vi "AlliGator Action Loop.vi"(8 "Error In":errorcluster) -> (0 "Error Out":errorcluster)   [LabVIEW 2021, in "AlliGator Action Engine.lvlib"]
doc: "AlliGator action dispatcher.\nEach action array is handled as a package, each action in the array being sent to the appropriate category (Files, Image, Phasor Graph, etc.)."
uses:
  AlliGator Action Engine.lvlib
  Internal Variables/AlliGator Internal Variables v2.ctl
  <vilib>/vision/Image Controls.llb/IMAQ Image.ctl
  Internal Variables/AlliGator Gate Image Set.ctl
  Files/AlliGator FLI Dataset Type.ctl
  Files/AlliGator Data Series Type.ctl
  Dual-Channel Datasets/AlliGator Dataset Channel.ctl
  Settings/AlliGator Gate Arithmetic.ctl
  Source Image/AlliGator Displayed Image.ctl
  Image/Named ROI Description.ctl
  Phasor Graph/AlliGator Decay Metadata v3.ctl
  Decay Analysis/Decay Preprocessing/AlliGator Decay Background Subtraction Info.ctl
  Decay Analysis/Decay Preprocessing/AlliGator Baseline Subtraction Method.ctl
  Graphs/XY Graph/XY Graph Plot Shift Parameters.ctl
  Graphs/XY Graph/XY Graph Plot Shift Method.ctl
  Decay Analysis/Decay Preprocessing/AlliGator Decay Extrapolation Parameters.ctl
  Phasor/Calibration Phasor (m, phi).ctl
  Phasor/Phasor Reference Series.ctl
  Phasor/Phasor Calibration Map v2.ctl
  Phasor/Phasor (g, s).ctl
  Phasor Graph/AlliGator Raw Phasor Plot Data v5.ctl
  Phasor/Phasor Standard Deviation Options.ctl
  Phasor Plot/AlliGator Phasor Multi-Harmonic Data.ctl
  Phasor/Phasor Harmonic Data.ctl
  Decay Fit Parameter Map/AlliGator Decay Fit Options & Parameters v4.ctl
  Fits/IRF(X)PSED/Decay Fit Options v4.ctl
  Fits/Decay Convolution/Decay Model.ctl
  Fits/Residual Type.ctl
  Fits/IRF(X)PSED/Fit Weights Type v2.ctl
  Fits/Non-linear Fitting Method v2.ctl
  Fits/Fit Calculation Method.ctl
  Fits/Non-linear Fitting Algorithm.ctl
  Decay Analysis/Decay Fit/AlliGator Decay Fit Parameter Constraints 2.ctl
  Fits/IRF(X)PSED/Decay Fit Parameters In List.ctl
  Fits/IRF(X)PSED/MLE Baseline Offset Type.ctl
  Decay Analysis/Decay Preprocessing/AlliGator Decay Preprocessing Parameters.ctl
  Fits/IRF(X)PSED/Decay Fit Parameters & Derived Quantities List v2.ctl
  Fits/IRF(X)PSED/Decay Fit Result Constraint.ctl
  Decay Fit Parameter Map/AlliGator Parameter Maps Data.ctl
  Globals, Variables, Constants/AlliGator Refnums List.ctl
  AlliGator Q Event.ctl
  Settings/AlliGator Settings List.ctl
  Graphs/XY Graph/XY Graph Selected Plot Info.ctl
  Graphs/XY Graph/XY Graph Refnum.ctl
  <vilib>/Utility/miscctls.llb/LVPoint32TypeDef.ctl
  Graphs/XY Graph/XY Graph Mouse Click Event Data.ctl
  Debug/AlliGator Debug Action List.ctl
  Alligator Elements Order in Action Stack.ctl
  bb653f8f-7323-4417-bc10-ef5a2241dee5.vi
  Globals, Variables, Constants/AlliGator Globals.vi
  Variant/Variant to Data/Variant to Boolean.vi
  AlliGator Add Action Array to Stack.vi
  Error/Error.lvlib
  Utilities/Utilities.lvlib
  GUI/AlliGator GUI.lvlib
  Notebook/Notebook.lvlib
  Globals, Variables, Constants/AlliGator Globals, Variables & Constants.lvlib
  Settings/AlliGator Settings.lvlib
  Graphs/XY Graph/XY Graph Add-Ons.lvlib
  Variant/Variant to Data/Variant to Data.lvlib
  Decay Fit Parameter Map/AlliGator Decay Fit Parameter Map.lvlib
  Debug/AlliGator Debug.lvlib
  Phasor/Phasor.lvlib
  Image/Image.lvlib
  Decay Analysis/Decay Preprocessing/AlliGator Decay Preprocessing.lvlib
  Phasor Graph/AlliGator Phasor Graph.lvlib
  Files/AlliGator Files.lvlib
  Internal Variables/AlliGator Internal Variables.lvlib
  Phasor Plot/AlliGator Phasor Plot.lvlib
  Source Image/AlliGator Source Image.lvlib
  Fits/Fits.lvlib
  Decay Analysis/Decay Fit/AlliGator Decay Fit.lvlib
  Python Plugins API/AlliGator Python Plugins.lvlib
  Dual-Channel Datasets/AlliGator Dual-Channel Datasets.lvlib
  Test Suites/AlliGator Test Suite.lvlib
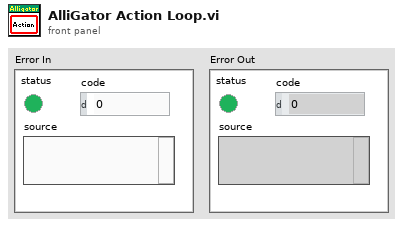
[diagram p1: front panel]
types:
  T1 = typedef "AlliGator Globals, Variables & Constants.lvlib/AlliGator Refnums List.ctl" = enum16{"---------- AlliGator Controls ----------", "AlliGator Tab Control Refnum", "---------- AlliGator Indicators ----------", "Source Image Display Refnum", "Phasor Plot Display Refnum", "Decay Fit Parameter Map Refnum", "---------- AlliGator VIs ----------", "AlliGator Refnum", "AlliGator Settings Refnum", "AlliGator Launcher Refnum"}
  T2 = typedef "AlliGator Internal Variables.lvlib/AlliGator Internal Variables v2.ctl" = cluster{"----------------------------- Images -----------------------------":u8, "Displayed Image":T3, "White Light Image":T3, "Mask Image":T3, "ROI Mask Image":T3, "Current Dataset Images 1":T4, "Background Dataset Images 1":T4, "Current Dataset Images 2":T4, "Background Dataset Images 2":T4, "Current Dataset Arithmetic Images":T4, "Accumulated Dataset Images 1":T4, "Accumulated Dataset Images 2":T4, "Accumulated Dataset Arithmetic Images":T4, "----------------------------- File Paths -----------------------------":u8, "Phasor Plot Image":T3, "Decay Fit Parameter Map Image":T3, "Parameter Map Image":T3, "Single Data Point Path":path, "White Light Image Path":path, "Mask Image Path":path, "Time-Series Folder":path, "[Time-Series Paths]":path[], "----------------------------- FLI Dataset -----------------------------":u8, "Current Dataset":i32, "Single Dataset Type":T5, "Current Folder":string, "AlliGator Data Series Type":T6, "# Datasets":i32, "Dual-Channel Dataset":bool, "Selected Channel Name":string, "Dataset Channel":T7, "Channel Arithmetic":T8, "Dual-Channel Background Dataset":bool, "Background Channel":T7, "Dual-Channel Accumulated Dataset":bool, "Start Time":dbl, "[Time-Series Timestamps]":dbl[], "[Intensity Corrections]":dbl[], "Time Series Script":bool, "Type of Displayed Image":T9, "Gate Image Slide":u16, "# Gates":i32, "ROIs":T10[], "----------------------------- Decays -----------------------------":u8, "ROI Decay":cluster{"t Array":dbl[], "I Array":dbl[]}, "Valid Decay":bool, "Decay  Metadata":T12, "Reference Decay Plot Name":string, "Reference Decay":cluster{"t Array":dbl[], "I Array":dbl[]}, "Decay Shift Plot":cluster{"Time Stamps":dbl[], "Decay Shifts":dbl[]}, "[Decays Max Values]":sgl[], "[Decays Min Values]":sgl[], "----------------------------- Calibration -----------------------------":u8, "Calibration Phasor":T18, "Calibration Phasor Series":T19, "Phasor Calibration Map":T20, "Calibration Map MD5 Digest":string, "----------------------------- Phasor Graph -----------------------------":u8, "Last Raw Phasor":T21, "Last Calibrated Phasor":T21, "Last Calibrated Phasor SDV":T21, "Phasor Graph:Phasor Plot":cluster{"g Array":dbl[], "s Array":dbl[]}, "Phasor Graph:Phasor SDV Plot":cluster{"g Array":dbl[], "s Array":dbl[]}, "[Phasor Graph:Raw Phasor Plots]":T22[], "Phasor Plot locked to Ref 1":i32, "[Phasor Plot(s) locked to Ref 1]":i32[], "[Phasor Plot(s) locked to Ref 2]":i32[], "[Pixel Phasors]":T21[], "----------------------------- Phasor Plot -----------------------------":u8, "[[Sum Image]]":dbl[][], "[[CSG Phasors]]":csg[][], "[[Valid Pixel?]]":bool[][], "[[Phasor Ratios]]":dbl[][], "[[Average Lifetimes]]":dbl[][], "Amplitude Weighted Average Lifetime":bool, "I/m/phi Dataset":cluster{"I/m/phi Dataset?":bool, "Base Frequency":dbl[unit], "Harmonic Orders":u8[]}, "Multi Phasor Plot Data":T24, "----------------------------- Decay Fit Parameter Map -----------------------------":u8, "Decay Fit Options & Parameters":T26, "Fit Options: Decay Preprocessing Parameters":T37, "Fit Options: Reference Decay":cluster{"t Array":dbl[], "I Array":dbl[]}, "Is Full Image Parameters Map":bool, "Is Single-Pixels Parameters Map":bool, "NLSF Parameters Map X Resolution":i32, "NLSF Parameters Map Y Resolution":i32, "[Single Decay Fit Parameters]":dbl[], "Fit Model":T28, "[[Multiple Decays Fit Parameters]]":dbl[][], "[[Multiple Decays Fit Parameter SDVs]]":dbl[][], "[[IRFs]]":dbl[][], "[ROI Descriptors]":T11[], "IRF Array Time Axis":dbl[], "Decay Array Time Axis":dbl[], "[Decay Fit Parameter Names]":T38[], "[Decay Sum]":dbl[], "Array of Decay Fit Result Constraints":T39[], "Selected ROIs Array":bool[], "----------------------------- Parameter Maps -----------------------------":u8, "[Map Set Names]":string[], "[Parameter Maps]":T40[], "[[User-defined Quantities]]":dbl[][], "User-defined Quantity":string}
  T3 = typedef "IMAQ Image.ctl" = refnum<image>
  T4 = typedef "AlliGator Internal Variables.lvlib/AlliGator Gate Image Set.ctl" = cluster{"SGL Gate Images":T3[], "SGL Sum Image":T3, "SGL Max Image":T3, "SGL Min Image":T3}
  T5 = typedef "AlliGator Files.lvlib/AlliGator FLI Dataset Type.ctl" = enum16{"HDF5 FLI Dataset", "Gate Image Folder", ".sdt FLI Dataset (Becker & Hickl)", ".ptu FLI Dataset (PicoQuant)", "SS1 FLI Dataset", "SS2 FLI Dataset", "I/m/phi Dataset", ".bin FLI Dataset (PicoQuant Binned)", ".bin FLI Dataset (Piccolo Binned)", ".mat FLI Dataset"}
  T6 = typedef "AlliGator Files.lvlib/AlliGator Data Series Type.ctl" = enum16{"Not a Supported Series", "Gate Images Folder Series", "SwissSPAD 2 Dataset Series", "B&H FLI Dataset Series", "PicoQuant PTU FLI Dataset Series", "PicoQuant BIN FLI Dataset Series", "Piccolo hist BIN FLI Dataset Series", "HDF5 FLI Dataset Series"}
  T7 = typedef "AlliGator Dual-Channel Datasets.lvlib/AlliGator Dataset Channel.ctl" = enum16{"G2", "INT"}
  T8 = typedef "AlliGator Settings.lvlib/AlliGator Gate Arithmetic.ctl" = enum16{"None", "INT-G2", "G2/INT*<INT>", "(1 - G2/INT)*<INT>"}
  T9 = typedef "AlliGator Source Image.lvlib/AlliGator Displayed Image.ctl" = enum16{"Single Gate", "Sum of All Gates", "Max of All Gates", "Min of All Gates", "-", "White Ligth Image", "Mask Image"}
  T10 = typedef "Image.lvlib/Named ROI Description.ctl" = cluster{"ROI Descriptor":T11, "ROI Name":string, "Overlay Color":u32}
  T11 = typedef "ROI Descriptor" = cluster{"Global Rectangle":i32[], "Contours":cluster{"ID":enum32{"External", "Internal"}, "Type":u32, "Coordinates":i32[]}[]}
  T12 = typedef "AlliGator Phasor Graph.lvlib/AlliGator Decay Metadata v3.ctl" = cluster{"ROI Descriptor":T11, "ROI Center":cluster{"X":i32, "Y":i32}, "Decay Background Subtraction Info":T13, "Decay Reverted":bool, "Decay Smoothened":bool, "Decay Straightened":bool, "Fitted Tau (Decay Straightening)":dbl, "Decay Shift Parameters":T15, "Decay Shifted":bool, "Decay Extrapolated":bool, "Decay Extrapolation Parameters":T17, "Decay Normalized":bool, "Fold Decay":bool, "# Folds":u32}
  T13 = typedef "AlliGator Decay Preprocessing.lvlib/AlliGator Decay Background Subtraction Info.ctl" = cluster{"Laser Period":dbl[unit], "Gate Duration":dbl[unit], "Baseline Subtraction Method":T14, "Background Definition Range":cluster{"Min Gate":dbl[unit], "Max Gate":dbl[unit]}, "Total Intensity w/o Bkgd Subtraction":dbl, "Bkgd-subtracted Intensity (exp)":dbl, "# Data Points":i32, "Background/Gate":dbl, "Fitted Lifetime":dbl[unit], "Bkgd-subtracted Intensity (theo)":dbl}
  T14 = typedef "AlliGator Decay Preprocessing.lvlib/AlliGator Baseline Subtraction Method.ctl" = enum16{"Mean", "Min", "Square Gated Single-Exponential", "File", "Constant"}
  T15 = typedef "XY Graph Add-Ons.lvlib/XY Graph Plot Shift Parameters.ctl" = cluster{"Type":T16, "Shift":dbl[unit], "Threshold":dbl, "Rotate":bool}
  T16 = typedef "XY Graph Add-Ons.lvlib/XY Graph Plot Shift Method.ctl" = enum16{"Default", "CFD", "Threshold", "Cross-Correlation"}
  T17 = typedef "AlliGator Decay Preprocessing.lvlib/AlliGator Decay Extrapolation Parameters.ctl" = cluster{"Additional Points":u32, "Head Fraction":dbl, "Fitted Tau":dbl, "Use Periodicity":bool, "Use Cursors":bool, "Tail Fraction":dbl}
  T18 = typedef "Phasor.lvlib/Calibration Phasor (m, phi).ctl" = cluster{"m":dbl, "phi":dbl, "Phasor Frequency":dbl[unit], "Reference Lifetime":dbl[unit]}
  T19 = typedef "Phasor.lvlib/Phasor Reference Series.ctl" = cluster{"m Array":dbl[], "phi Array":dbl[], "Phasor Frequency":dbl[unit], "Calibration Lifetime":dbl[unit]}
  T20 = typedef "Phasor.lvlib/Phasor Calibration Map v2.ctl" = cluster{"Phasor Frequency":dbl[unit], "Calibration Lifetime":dbl[unit], "ROI Centers":cluster{"X":i32, "Y":i32}[], "ROI Descriptors":T11[], "Map Resolution X":i32, "Map Resolution Y":i32, "z Array":cdb[]}
  T21 = typedef "Phasor.lvlib/Phasor (g, s).ctl" = cluster{"g":dbl, "s":dbl}
  T22 = typedef "AlliGator Phasor Graph.lvlib/AlliGator Raw Phasor Plot Data v5.ctl" = cluster{"Phasor Plot Name":string, "Raw Phasor Plot":T21[], "Phasor Frequency":dbl[unit], "[Decay Metadata]":T12[], "Raw Phasor Plot SDV":T21[], "Phasor SDV Options":T23, "[Calibration Phasor]":T18[], "Intensity Array":dbl[]}
  T23 = typedef "Phasor.lvlib/Phasor Standard Deviation Options.ctl" = cluster{"Compute Estimated SDV":bool, "# Replicas":u32, "Use Estimated Average Phasor":bool}
  T24 = typedef "AlliGator Phasor Plot.lvlib/AlliGator Phasor Multi-Harmonic Data.ctl" = cluster{"Base Frequency":dbl[unit], "# Harmonics":u8, "Harmonic Orders":u8[], "Phasor Plot Settings Checksum":u64, "Phasor Harmonic Data Array":T25[]}
  T25 = typedef "Phasor.lvlib/Phasor Harmonic Data.ctl" = cluster{"Phasor Harmonic Name":string, "Phasor Plot Settings Checksum":u64, "Phasor Frequency":dbl[unit], "Base Frequency":dbl[unit], "Harmonic Order":u8, "Phasor Plot Parameters":string, "Phasor Array [[CSG]]":csg[][], "Dataset File Path":path}
  T26 = typedef "AlliGator Decay Fit Parameter Map.lvlib/AlliGator Decay Fit Options & Parameters v4.ctl" = cluster{"SYNC Period":dbl[unit], "Fit Options":T27, "Fit Parameter Constraints":T34[], "MLE Baseline Offset":dbl, "MLE Baseline Offset Type":T36}
  T27 = typedef "Fits.lvlib/Decay Fit Options v4.ctl" = cluster{"Show Fit Residuals":bool, "Fit Model":T28, "Residual Type":T29, "Max Decay Percentile":dbl, "Min Decay Percentile":dbl, "Show Full Decay":bool, "Weights":T30, "Fitting Method":T31, "Compute Parameter Uncertainties":bool, "Periodic Boundaries":bool, "Model Calculation":T32, "Period":dbl[unit], "Termination Criteria":cluster{"Max Iterations":i32, "Max Function Calls":i32, "Max Time":dbl[unit], "Function Tolerance":dbl, "Parameter Tolerance":dbl, "Gradient Tolerance":dbl, "Min Lambda":dbl, "Max Lambda":dbl, "Initial Tick Count":u32}, "Offset Resolution":dbl[unit], "Use Local IRF":bool, "Fitting Algorithm":T33, "Show Confidence Interval ":bool, "Confidence Level":dbl}
  T28 = typedef "Fits.lvlib/Decay Model.ctl" = enum16{"1-Exponential", "2-Exponentials"}
  T29 = typedef "Fits.lvlib/Residual Type.ctl" = enum16{"Standard", "Normalized", "Reduced"}
  T30 = typedef "Fits.lvlib/Fit Weights Type v2.ctl" = enum16{"Unweighted", "1/Variance (Neyman)", "1/Variance (Pearson)", "Best of All"}
  T31 = typedef "Fits.lvlib/Non-linear Fitting Method v2.ctl" = enum16{"Least Square", "Least Absolute Residual", "Bisquare", "MLE", "-", "Best of All"}
  T32 = typedef "Fits.lvlib/Fit Calculation Method.ctl" = enum16{"Simulation", "Convolution", "Integration"}
  T33 = typedef "Fits.lvlib/Non-linear Fitting Algorithm.ctl" = enum16{"Levenberg-Marquardt", "Trust-Region Dogleg"}
  T34 = typedef "AlliGator Decay Fit.lvlib/AlliGator Decay Fit Parameter Constraints 2.ctl" = cluster{"Fit Parameter":T35, "Min Value":dbl, "Max Value":dbl, "Global":bool, "Used":bool}
  T35 = typedef "Fits.lvlib/Decay Fit Parameters In List.ctl" = enum16{"Offset", "Baseline", "A_1", "tau_1", "A_2", "tau_2"}
  T36 = typedef "Fits.lvlib/MLE Baseline Offset Type.ctl" = enum32{"Absolute", "Percentage"}
  T37 = typedef "AlliGator Decay Preprocessing.lvlib/AlliGator Decay Preprocessing Parameters.ctl" = cluster{"Background Subtraction":bool, "Straighten Decay":bool, "Reverse Gates":bool, "1-Normalized Decay":bool, "Smoothen Decay":bool, "Smoothing Parameter":dbl, "Shift Decay":bool, "Decay Shift Parameters":T15, "Extrapolate Decay":bool, "Additional Points":u32, "Head Fraction":dbl, "Pixel-Normalize Decay":bool, "Use Periodicity":bool, "Use Cursors":bool, "Tail Fraction":dbl, "Use Decay Pre-Processing":bool, "Fold Decay":bool, "# Folds":u32, "[0-1]-Normalized Decay":bool}
  T38 = typedef "Fits.lvlib/Decay Fit Parameters & Derived Quantities List v2.ctl" = enum16{"Offset", "Baseline", "A_1", "tau_1", "A_2", "tau_2", "<tau>_a", "f1_a", "f2_a", "<tau>_i", "f1_i", "f2_i", "-", "R^2", "Chi^2"}
  T39 = typedef "Fits.lvlib/Decay Fit Result Constraint.ctl" = cluster{"Fit Parameter":enum16{"Offset", "Baseline", "A_1", "tau_1", "A_2", "tau_2", "<tau>_a", "f1_a", "f2_a", "<tau>_i", "f1_i", "f2_i", "-", "R^2", "Chi^2", "Max Relative Residual", "<Residual ACF>", "Residual ACF SDV", "tau_2/tau_1"}, "Min Value":dbl, "Max Value":dbl, "Use Constraint":bool}
  T40 = typedef "AlliGator Decay Fit Parameter Map.lvlib/AlliGator Parameter Maps Data.ctl" = cluster{"Map Set Name":string, "[Parameter Names]":string[], "[[Parameters]]":dbl[][], "[[Parameter SDVs]]":dbl[][], "Decay Array Time Axis":dbl[], "[[IRFs]]":dbl[][], "IRF Array Time Axis":dbl[], "X Resolution":i32, "Y Resolution":i32, "Intensity Array":dbl[]}
  T41 = typedef "AlliGator Action Engine.lvlib/AlliGator Q Event.ctl" = enum16{"---- Files ----", "Files:Set Batch Export Files To Save", "Files:Set Dataset Loading & Pre-processing Options", "Files:Check #Frames in Dataset", "Files:Increment Frame Index", "Files:Open Mask Image", "Files:Open White Light Image", "Files:Open Single Dataset", "Files:New Folder of Folders Selected", "Files:Load File (all Types)_Scriptable", "Files:Move Flattened Series to Folders Series", "Files:Select Folder", "Files:Load FLI Dataset", "Files:Load Swiss SPAD 1 Dataset", "Files:Load Swiss SPAD 2 Dataset", "Files:Load .sdt FLI Dataset", "Files:Load .ptu FLI Dataset", "Files:Load .bin FLI Dataset", "Files:Load Single Gate Image Folder", "Files:Load I/m/phi Dataset (deprecated)", "Files:Load Single Image", "Files:Subtract Background File", "Files:Export FLI Dataset", "Files:Load HDF5 FLI Dataset", "Files:Set Destination File Path", "Files:Save Mask Image", "Files:Batch Conversion", "Files:New Folder Selected", "Files:Close FLI Dataset", "Files:Close FLI Dataset Series", "Files:Close White Light Image", "Files:Close Mask Image", "---- FLI Dataset ----", "FLI Dataset:Channel Arithmetic", "FLI Dataset:Export Average Lifetime Map as ASCII", "FLI Dataset:Export User-Defined Quantity Map as ASCII", "FLI Dataset:Python Function FLI Dataset Event", "FLI Dataset:ROI Analysis", "FLI Dataset:Tilted Logistic Square Gated IRF Characteristics Map", "FLI Dataset:Logistic Square Gated IRF Characteristics Map", "FLI Dataset:Square Gated IRF Characteristics Map", "FLI Dataset:Multi-ROI Single-Pixel Phasor Analysis", "FLI Dataset:Multi-ROI Single-Pixel NLSF Analysis", "FLI Dataset:All ROIs IRF Extraction", "FLI Dataset:All ROIs Decay Fit Non-Interactive (Fast + Individual IRF)", "FLI Dataset:All ROIs Phasor Analysis", "FLI Dataset:All ROIs Decay Fit", "FLI Dataset:Fluorescence Decay Statistics", "FLI Dataset:Update Decay Statistics Graph", "FLI Dataset:Get Decay from ROI", "FLI Dataset:All ROIs Average Lifetimes", "FLI Dataset:Save/Load Local IRFs", "FLI Dataset:Clear Local IRFs", "FLI Dataset:Phasor Calibration Maps (# Gates Series) Script", "FLI Dataset:Calibrated Phasor Map Series", "---- FLI Dataset Series ----", "FLI Dataset Series:Sum All Datasets in Series", "FLI Dataset Series:Add Dataset to Accumulated Dataset", "FLI Dataset Series:Display Accumulated Dataset", "FLI Dataset Series:Clear Dataset Series Sum", "FLI Dataset Series:Time-Series Analysis (NLSF)", "FLI Dataset Series:Time-Series Analysis (Phasor)", "---- Image ----", "Image:Update Image Profile Plots", "Image:Image Histogram Cursor Move", "Image:Image Histogram", "Image:Image Contrast", "Image:Set Image Histogram Cursor Move Flag", "Image:Clear Image Overlay", "Image:Use ROI as Search Area", "Image:Set ROI Diameter", "Image:Save Image Data as TIFF", "Image:Save Displayed Image with Overlay", "Image:Save Image Overlay Only", "Image:Save Image as Hot Pixel Mask", "Image:Change Source Image Color Palette", "Image:Copy Image to Clipboard", "Image:Source Image ROI Selection", "Image:Delete All ROIs", "Image:Delete All Unselected ROIs", "Image:Delete ROI", "Image:Merge All ROIs", "Image:Store ROI", "Image:Source Image ROI Storage", "Image:Export ROI Description to Notebook", "Image:Save ROI", "Image:Load ROI", "Image:Paste ROI Definition", "Image:Clear ROI", "Image:Identify ROIs in Mask Image", "Image:Create Complementary ROI", "Image:Create Contour ROI", "Image:Create ROI(s) from Pixels with Peak above Min_Scriptable", "Image:Create ROI(s) from Pixels with Intensity above Min_Scriptable", "Image:Compute ROI Statistics", "Image:Delete ROI(s) based on ROI Characteristics", "Image:Create ROI Grid", "Image:ROI to Individual Pixel ROIs", "Image:Python Function Source Image Event", "Image:Show Phasor Calibration Map ROI Centers", "Image:Convert ROI to Mask Image", "Image:Mouse Move", "Image:Mouse Up", "Image:Set Source Image Mouse Move Flag", "Image:Add Scale Bar Overlay", "Image:Delete Existing ROIs Option", "Image:Overlay ROI Median", "Image:Check Current ROI", "Image:Update True Pixel Value", "---- Decay ----", "Decay:Clear IRF/Reference Plot", "Decay:Add Decay to Graph", "Decay:Smoothen Plot", "Decay:Smoothen Plot Tail", "Decay:Average Selected Plots", "Decay:Extract IRF", "Decay:Optimal IRF Extraction", "Decay:Threshold IRF", "Decay:Fit to Model IRF", "Decay:Fit IRF to Square Gate", "Decay:Fit IRF to Logistic Square Gate", "Decay:Fit IRF to Tilted Logistic Square Gate", "Decay:Create Bounding Cursors Set", "Decay:Export Bounding Cursors Definition to Notebook", "Decay:Denoise Plot", "Decay:Compute Cumulative Function", "Decay:Use as Reference Decay", "Decay:Show Reference Decay/IRF", "Decay:Extrapolate Decay", "Decay:Create Head & Tail Bounding Cursors", "Decay:Store Cursor-defined Head & Tail Fractions", "Decay:Rebin Plot", "Decay:1-Normalize Decay", "Decay:[0-1]-Normalize Plot", "Decay:Straighten Decay", "Decay:Shift Decay", "Decay:Fold Decay", "Decay:Fit Decay", "Decay:Global Fit of Selected Decays", "Decay:Post Global Fit Script", "Decay:Add Global Fit Parameters to Graph", "Decay:Add Decay Parameter(s) to Plot (Graph)", "Decay:Export Decay to Phasor Graph", "Decay:Compute Average Lifetime", "Decay:Plot Convolution", "Decay:Graph Tip Strip Update", "---- Decay Statistics ----", "Decay Statistics:Tip Strip Update", "---- Intensity Time Trace ----", "Intensity Time Trace:Use File Timestamp", "Intensity Time Trace:Load Intensity Corrections File", "Intensity Time Trace:Clear Intensity Corrections File", "Intensity Time Trace:Tip Strip Update", "---- Phasor Plot ----", "Phasor Plot:Build Phasor Plot", "Phasor Plot:Change Phasor Plot Color Palette", "Phasor Plot:Adjust Phasor Plot Display Range", "Phasor Plot:Highlight Image ROI in Phasor Plot", "Phasor Plot:Save Phasor Plot Image with Overlay", "Phasor Plot:Export Complex Phasor Map", "Phasor Plot:Export Phasor Ratio Map", "Phasor Plot:Export Average Lifetime Map", "Phasor Plot:Compute Phase Lifetime Histogram", "Phasor Plot:Compute Phasor Ratio Histogram", "Phasor Plot:Compute Phase Lifetime vs Intensity Scatter Plot", "Phasor Plot:Weber 2-Component Decomposition", "Phasor Plot:Update Phasor Color Map Vertices", "Phasor Plot:Clear Phasor Overlay", "Phasor Plot:Use Segment Extremities as References", "Phasor Plot:Use UC/Segment Intersections as References", "Phasor Plot:Use UC/Principal Axis Intersections as References", "Phasor Plot:Use UC/Linear Fit Intersections as References", "Phasor Plot:Update Phasor Plot Reference", "Phasor Plot:Show Local Phasor Info in Phasor Plot", "Phasor Plot:Update Phasor Plot State", "Phasor Plot:Phasor Plot ROI Storage", "Phasor Plot:Phasor Plot ROI Selection", "Phasor Plot:Python Function Phasor Plot Event", "Phasor Plot:Overlay Phasor ROI, Ratio or Map in Source Image", "Phasor Plot:Compute Decay of Selected Phasors", "Phasor Plot:Phasor at Image Pixel", "Phasor Plot:Mouse Move", "Phasor Plot:Mouse Up", "Phasor Plot:Display Range Mouse Move", "Phasor Plot:Set Mouse Move Flag", "Phasor Plot:Update True Phasor Plot Value", "---- Phasor Graph ----", "Phasor Graph:Get Phasor Value", "Phasor Graph:Create New Phasor Plot Dialog", "Phasor Graph:Update Last Phasor Value", "Phasor Graph:Update Phasor (m, phi)", "Phasor Graph:Remove Single Phasor from Plot", "Phasor Graph:Add Single Phasor to Plot", "Phasor Graph:Remove Phasor Plot", "Phasor Graph:Remove Selected Phasor Plots", "Phasor Graph:Clear Phasor Data", "Phasor Graph:Clear Phasor Graph", "Phasor Graph:Cursor Move", "Phasor Graph:Draw Cursor Connecting Line", "Phasor Graph:Clear Cursor Connecting Line", "Phasor Graph:Find UC Intersection", "Phasor Graph:Use UC/Cursor-Defined Line Intersections", "Phasor Graph:Use Selected Plots Fitted Line/UC Intersections", "Phasor Graph:Use Selected Plots Principal Axis/UC Intersections", "Phasor Graph:Show Single Phasor", "Phasor Graph:Save Single Phasor Plot", "Phasor Graph:Save All Phasor Plots", "Phasor Graph:Load Phasor Plot(s)", "Phasor Graph:Phasor Multiplication", "Phasor Graph:Compute Average Phasor", "Phasor Graph:Compute Multiple Average Phasors (Selected Plots)", "Phasor Graph:Export Single Phasor Plot Phase Lifetimes", "Phasor Graph:Parameter 2 vs Parameter 1 Scatter Plot", "Phasor Graph:Use Cursor n Location", "Phasor Graph:Set Reference n to Current Phase Lifetime Value", "Phasor Graph:Set Reference n to Lifetime Value", "Phasor Graph:Set Cursor n Location", "Phasor Graph:Save Phasor Graph Image", "Phasor Graph:Update SEPL Plot", "Phasor Graph:Export Single Phasor Plot Data", "Phasor Graph:Export Selected Phasor Plots Data", "Phasor Graph:Python Function Phasor Graph Event", "Phasor Graph:Tip Strip Update", "---- Calibration ----", "Calibration:Set Calibration Type", "Calibration:Load/Save Phasor Calibration", "Calibration:Load/Save Phasor Calibration Series", "Calibration:Load/Save Phasor Calibration Map", "Calibration:Use as Calibration", "Calibration:Compute Optimal Calibration from Phasor References", "Calibration:Clear Phasor Calibration", "Calibration:Single Phasor Calibration Information", "Calibration:Use as Calibration Series", "Calibration:Use as Calibration Map", "Calibration:Clear Calibration Series", "Calibration:Phasor Calibration Series Information", "Calibration:Clear Calibration Map", "Calibration:Phasor Calibration Map Information", "Calibration:Apply Phasor Calibration", "Calibration:Update Single Plot Calibration", "Calibration:Update Multiple Plots Calibration", "Calibration:Clear Single Plot Calibration", "Calibration:Clear All Plots Calibrations", "Calibration:Clear Plot(s) Calibration(s)?", "---- Phasor Ratio ----", "Phasor Ratio:Clear Reference n", "Phasor Ratio:Toggle Selected Plot(s)  Lock to Reference 1", "Phasor Ratio:Use as Reference n", "Phasor Ratio:Send Reference n to Notebook", "Phasor Ratio:Toggle Selected Plot(s)  Lock to Reference 2", "Phasor Ratio:Compute Phasor Ratio at Mouse Location", "Phasor Ratio:Compute Phasor Plot's Average Phasor Ratio", "Phasor Ratio:Compute Time-Series Phasor Ratios", "Phasor Ratio:Fit Line to Phasor Ratio Plot", "Phasor Ratio:Save References", "Phasor Ratio:Load References", "Phasor Ratio:Update Phasor Reference 1", "Phasor Ratio:Update Phasor Reference 2", "Phasor Ratio:Move Cursor n to Reference n", "Phasor Ratio:Use as Phasor Reference 1 Lifetime", "Phasor Ratio:Use as Phasor Reference 2 Lifetime", "Phasor Ratio:Export Phasor Ratio Map as ASCII", "Phasor Ratio:Tip Strip Update", "---- Lifetime & Other Parameters Graph ----", "Lifetime:Compute Sliced Mean, SDV and CV Plots", "Lifetime:Plot Decay Shifts", "Lifetime:Plot Histogram", "---- Decay Fit Parameter Map ----", "Decay Fit Parameter Map:Export ROI NLSF Data as ASCII", "Decay Fit Parameter Map:Set Decay Fit Parameter Map Selection", "Decay Fit Parameter Map:Build Decay Fit Parameter Map", "Decay Fit Parameter Map:Change Decay Fit Parameter Map Color Palette", "Decay Fit Parameter Map:Export Decay Fit Parameter Map Data as ASCII", "Decay Fit Parameter Map:Export All Decay Fit Parameter Maps Data as ASCII", "Decay Fit Parameter Map:Selected Parameter Scatterplot", "Decay Fit Parameter Map:Parameter 2 vs Parameter 1 Scatterplot", "Decay Fit Parameter Map:Save Decay Fit Parameter Map Image", "Decay Fit Parameter Map:Save-Load IRFs & Fit Data", "Decay Fit Parameter Map:Update Local Decay Plots", "Decay Fit Parameter Map:Python Function Decay Fit Parameters Map Event", "Decay Fit Parameter Map:Overlay Decay Fit Parameter Map in Source Image", "Decay Fit Parameter Map:Selected Parameter vs Intensity Scatterplot", "Decay Fit Parameter Map:Mouse Up", "Decay Fit Parameter Map:Mouse Move", "Decay Fit Parameter Map:Display Range Mouse Move", "Decay Fit Parameter Map:Change Map Resolution", "Decay Fit Parameter Map:Variance Significance Maps", "Decay Fit Parameter Map:Fit Result Constraints Window", "---- Parameter Map ----", "Parameter Map:Export ROI Parameters Data as ASCII", "Parameter Map:Add Parameter Map Set", "Parameter Map:Delete Parameter Map Set", "Parameter Map:Update Parameter List", "Parameter Map:Build Parameter Map", "Parameter Map:Change Parameter Map Color Palette", "Parameter Map:Export Parameter Map Data as ASCII", "Parameter Map:Export All Parameter Maps Data as ASCII", "Parameter Map:Selected Parameter Scatterplot", "Parameter Map:Parameter 2 vs Parameter 1 Scatterplot", "Parameter Map:Selected Parameter vs Intensity Scatterplot", "Parameter Map:Save Parameter Map Image", "Parameter Map:Save-Load IRFs & Parameter Maps (TODO)", "Parameter Map:Set Parameter Map Selection", "Parameter Map:Python Function Parameter Map Event", "Parameter Map:Overlay Parameter Map in Source Image", "Parameter Map:Update Local Decay Plots", "Parameter Map:Mouse Up", "Parameter Map:Mouse Move", "Parameter Map:Display Range Mouse Move", "---- Generic Graph ----", "Generic Graph:Generic XY Graph Event", "Generic Graph:Python Function XY Graph Event", "Generic Graph:New Plot", "Generic Graph:Save Plot", "Generic Graph:XY Plot Histogram", "Generic Graph:Set XY Graph Plot Name", "Generic Graph:Set Last Cursor Style", "Generic Graph:Tip Strip Update", "---- GUI ----", "GUI:Start Script", "GUI:Type of Displayed Image Changed", "GUI:Gate Image Slide Changed", "GUI:Show Busy Icon", "GUI:Show Busy Icon & Abort Button", "GUI:Hide Busy Icon", "GUI:Hide Busy Icon & Abort Button", "GUI:Abort", "GUI:End Script", "GUI:Start Timing", "GUI:End Timing", "GUI:Set State Indicator", "GUI:Send Parameters JSON Strings to Clipboard", "GUI:Set Gate Step", "GUI:Idle", "GUI:Initialization", "GUI:Quit", "GUI:Increment Dataset Index", "GUI:Set Dataset Index to -1", "GUI:Time Series Slider Moved", "GUI:Time Series Slider Changed", "GUI:Toggle Playback or Loop", "GUI:Playback Script", "GUI:Set Phasor Frequency", "GUI:Open Window", "GUI:Start Test Script", "GUI:End Test Script", "GUI:Set Verbose Mode", "GUI:Set Verbose Settings Mode", "DEBUG"}
  T42 = typedef "AlliGator GUI.lvlib/AlliGator Ctrl Refnums.ctl" = cluster{"Other AlliGator Ctrl Refnums":T43, "Phasor Plot Ctrl Refnums":T44, "Phasor Graph Ctrl Refnums":T45, "Dataset Control Refnums":T46, "Registered Events Ctrl Refnums":T47, "Image Histogram Ctrl Refnums":T48, "Decay Fit Map Ctrl Refnums":T49, "Parameter Map Ctrl Refnums":T50}
  T43 = typedef "AlliGator GUI.lvlib/AlliGator Other Ctrl Refnums.ctl" = cluster{"State Indicators":refnum<vi>, " Progress Bar":refnum<vi>, "Decay Graph Active":refnum<vi>, "Decay Statistics Bin":refnum<vi>, "Time Step":refnum<vi>, "Use File Timestamp":refnum<vi>, "Tab Control":refnum<vi>, "CPU":refnum<vi>, "Abort Fit":refnum<vi>, "Dataset File/Folder Path":refnum<vi>, "Abort ROI Creation":refnum<vi>, "Event LED":refnum<vi>, "Dataset File/Folder Path 2":refnum<vi>, "Dataset File/Folder Path 3":refnum<vi>, "Dataset File/Folder Path 4":refnum<vi>, "Dataset File/Folder Path 5":refnum<vi>, "Dataset File/Folder Path 6":refnum<vi>, "Dataset File/Folder Path 7":refnum<vi>, "Dataset File/Folder Path 8":refnum<vi>, "Dataset File/Folder Path 9":refnum<vi>, "Dataset File/Folder Path 10":refnum<vi>, "Dataset File/Folder Path 11":refnum<vi>}
  T44 = typedef "AlliGator GUI.lvlib/AlliGator Phasor Plot Ctrl Refnums.ctl" = cluster{"Phasor Ratio":refnum<vi>, "Modulus Lifetime":refnum<vi>, "Phasor at cursor (m, phi)":refnum<vi>, "Phase Lifetime":refnum<vi>, "Phasor at cursor (g, s)":refnum<vi>, "Phasor Plor Average Lifetime":refnum<vi>, "Phasor Plot Active":refnum<vi>, "Save Phasor Plot":refnum<vi>, "Image Overlay Color":refnum<vi>, "Phasor Plot Color Scale":refnum<vi>, "Reference 1 Button":refnum<vi>, "Reference 2 Button":refnum<vi>, "True Phasor Plot Value":refnum<vi>}
  T45 = typedef "AlliGator GUI.lvlib/AlliGator Phasor Graph Ctrl Refnums.ctl" = cluster{"Phasor Ratio":refnum<vi>, "Modulus Lifetime":refnum<vi>, "Phasor at cursor (m, phi)":refnum<vi>, "Phase Lifetime":refnum<vi>, "Phasor at cursor (g, s)":refnum<vi>, "Phasor Graph Average Lifetime":refnum<vi>, "Phasor Graph Active":refnum<vi>, "Save Phasor Graph":refnum<vi>, "Phasor Frame Slide":refnum<vi>, "Single Step Phasor":refnum<vi>, "Calibration Type":refnum<vi>, "Show Line":refnum<vi>, "Phase Lifetime 1":refnum<vi>, "Phase Lifetime 2":refnum<vi>, "Phasor Graph Frequency":refnum<vi>, "Phasor Reference 1 Control":refnum<vi>, "Phasor Reference 2 Control":refnum<vi>, "Calibration Lifetime":refnum<vi>, "Phase Lifetime SDV":refnum<vi>, "Average Lifetime SDV":refnum<vi>, "Phasor Ratio SDV":refnum<vi>, "Modulus Lifetime SDV":refnum<vi>}
  T46 = typedef "AlliGator GUI.lvlib/AlliGator Dataset Ctrl Refnums.ctl" = cluster{"Current Data":refnum<vi>, "Gate Image Slide":refnum<vi>, "Time Point Slide":refnum<vi>, "Current Time Stamp":refnum<vi>, "Save Image":refnum<vi>, "Displayed Image":refnum<vi>, "Overlay Mode":refnum<vi>, "Phasor Overlay Color":refnum<vi>, "Image Color Scale":refnum<vi>, "Use ROI as Search Area":refnum<vi>, "Source Image ROI Color":refnum<vi>, "True Pixel Value":refnum<vi>}
  T47 = typedef "AlliGator GUI.lvlib/AlliGator Registered Events Ctrl Refnums.ctl" = cluster{"Time Point Slider":refnum<vi>, "Phasor Plot Display Range":refnum<vi>, "Decay Graph":refnum<vi>, "Decay Statistics Graph":refnum<vi>, "Intensity Time Trace":refnum<vi>, "Phasor Graph":refnum<vi>, "Phasor Ratio Graph":refnum<vi>, "Lifetime Graph":refnum<vi>, "Phasor Plot Display":refnum<vi>, "Source Image Display":refnum<vi>, "Decay Fit Parameter Map Display Range":refnum<vi>, "Decay Fit Parameter Map Display":refnum<vi>, "Parameter Map Display Range":refnum<vi>, "Parameter Map Display":refnum<vi>, "Phasor Plot Display Range":refnum<vi>}
  T48 = typedef "AlliGator GUI.lvlib/AlliGator Image Histogram Control Refnums.ctl" = cluster{"Image Histogram":refnum<vi>, "Image Histogram Options":refnum<vi>, "Image Histogram Active":refnum<vi>, "Image Histogram Upper Percentile":refnum<vi>, "Image Histogram Lower Percentile":refnum<vi>, "Auto-Adjust Contrast":refnum<vi>}
  T49 = typedef "AlliGator Decay Fit Parameter Map.lvlib/AlliGator Decay Fit Map Control Refnums.ctl" = cluster{"Decay Fit Parameter Map Color Scale":refnum<vi>, "Decay Fit Parameter":refnum<vi>, "Max Parameter":refnum<vi>, "Min Parameter":refnum<vi>, "Decay Fit Parameter Map Display":refnum<vi>, "Decay Fit Parameter Map Display Range":refnum<vi>, "Decay Parameter Map X":refnum<vi>, "Decay Parameter Map Y":refnum<vi>, "Decay Parameter Map Value":refnum<vi>}
  T50 = typedef "AlliGator Parameter Map.lvlib/AlliGator Parameter Map Control Refnums.ctl" = cluster{"Parameter Map Color Scale":refnum<vi>, "Map Parameter":refnum<vi>, "Max Parameter":refnum<vi>, "Min Parameter":refnum<vi>, "Parameter Map Display":refnum<vi>, "Parameter Map Display Range":refnum<vi>, "Parameter Map Set":refnum<vi>, "Parameter Map X":refnum<vi>, "Parameter Map Y":refnum<vi>, "Parameter Map Value":refnum<vi>}
  T51 = typedef "XY Graph Add-Ons.lvlib/XY Graph Mouse Click Event Data.ctl" = cluster{"Multiplot XY Graph":T52, "Mouse Coordinates":T53}
  T52 = typedef "XY Graph Add-Ons.lvlib/XY Graph Refnum.ctl" = refnum<vi>
  T53 = typedef "LVPoint32TypeDef.ctl" = cluster{"Horizontal":i32, "Vertical":i32}
  T54 = typedef "XY Graph Add-Ons.lvlib/XY Graph Selected Plot Info.ctl" = cluster{"Multiplot XY Graph":T52, "Mouse Coordinates":T53, "Plot Index":i32}
  T55 = typedef "AlliGator Settings.lvlib/AlliGator Settings List.ctl" = enum16{"GUI:Visible Settings Tab", "GUI:Last Run Version", "Source Image:Use Image Histogram for Contrast", "Source Image:Low Count Pixels Rejection Options", "Source Image:High Count Pixels Rejection Options", "Source Image:Use Image Brightness", "Source Image:Blend Overlay with Image Background", "Source Image:Use Fixed ROI Diameter", "Source Image:ROI Diameter", "Source Image:ROI Center Color", "Source Image:Peak Threshold", "Source Image:Intensity Threshold", "Source Image:Image Binning Options", "Source Image:Image Smoothing Options", "Source Image:Image Histogram Active", "Source Image:Invert Binary Mask", "Source Image:Hot Pixel Removal", "Source Image:Overlay Analyzed ROI Center", "Source Image:Auto-Adjust Contrast", "Source Image:Histogram Lower Percentile", "Source Image:Histogram Upper Percentile", "Source Image:Save Source Image", "Source Image:Scale Bar Options", "Source Image:Image Resolution (Pixel Size)", "Source Image:Flatfield Correction", "Source Image:Show Dead Left Columns Correction", "Source Image:Dead Left Columns Correction", "Source Image:Image Pre-Processing Operations Order", "Source Image:Overlay ROI Median", "Source Image:Median Overlay Color", "Data Information:Gate Width", "Data Information:Nanotime Gate Separation", "Data Information:Macrotime Gate Separation", "Data Information:Gate Step", "Data Information:# Gates", "Data Information:Gate Image Exposure", "Data Information:Gate Image Integration", "Data Information:Gates to Skip", "Data Information:Gates to Keep", "Data Information:Define Gates to", "Data Information:Channel Name", "Data Information:Available Channel Names", "Data Information:Channel Arithmetic", "Data Information:Background File Subtraction", "Data Information:Background File", "Data Information:Background Scaling Factor", "Data Information:Background Pile-up Correction", "Data Information:Background Pixel Well Capacity", "Data Information:Laser Period", "Data Information:SYNC Period", "Data Information:Pile-up Correction", "Data Information:Pixel Well Capacity", "Data Information:Dataset Scaling Factor", "Fluorescence Decay_Decay Pre-Processing:Reverse Gates", "Fluorescence Decay_Decay Pre-Processing:Verbose Decay Pre-Processing", "Fluorescence Decay_Decay Pre-Processing:Use Decay Pre-Processing", "Fluorescence Decay_Decay Pre-Processing:Background Subtraction", "Fluorescence Decay_Decay Pre-Processing:Background Definition Range", "Fluorescence Decay_Decay Pre-Processing:Baseline Subtraction Method", "Fluorescence Decay_Decay Pre-Processing:Decay Pre-Processing Operations Order", "Fluorescence Decay_Decay Pre-Processing:Smoothing Parameter", "Fluorescence Decay_Decay Pre-Processing:Shift Decay", "Fluorescence Decay_Decay Pre-Processing:Decay Shift Parameters", "Fluorescence Decay_Decay Pre-Processing:Fold Decay", "Fluorescence Decay_Decay Pre-Processing:# Folds", "Fluorescence Decay_Decay Pre-Processing:1-Normalize Decay", "Fluorescence Decay_Decay Pre-Processing:[0-1]-Normalize Decay", "Fluorescence Decay_Decay Pre-Processing:Smoothen Decay", "Fluorescence Decay_Decay Pre-Processing:Extrapolate Decay", "Fluorescence Decay_Decay Pre-Processing:Use Periodicity", "Fluorescence Decay_Decay Pre-Processing:Use Cursors", "Fluorescence Decay_Decay Pre-Processing:Tail Fraction", "Fluorescence Decay_Decay Pre-Processing:Head Fraction", "Fluorescence Decay_Decay Pre-Processing:Additional Points", "Fluorescence Decay_Decay Pre-Processing:Straighten Decay", "Fluorescence Decay_Decay Pre-Processing:Constant Background", "Fluorescence Decay_Decay Pre-Processing:Pixel-Normalize Decay", "Fluorescence Decay_Advanced Analysis:Extract IRF instead of Decay", "Fluorescence Decay_Advanced Analysis:IRF Extraction Options", "Fluorescence Decay_Advanced Analysis:IRF Optimization Options", "Fluorescence Decay_Advanced Analysis:Square Pulse Options", "Fluorescence Decay_Advanced Analysis:IRF Order", "Fluorescence Decay_Advanced Analysis:IRF Time Constants", "Fluorescence Decay_Advanced Analysis:Wavelet Analysis Options", "Fluorescence Decay_Advanced Analysis:Average Lifetime Options", "Fluorescence Decay_Fit Options:Fit Options", "Fluorescence Decay_Fit Options:Use Legacy Fitting Approach", "Fluorescence Decay_Fit Options:Use Data Information Laser Period", "Fluorescence Decay_Fit Parameters:Displayed Fit Parameters", "Fluorescence Decay_Fit Parameters:Fit Parameter Constraints", "Fluorescence Decay_Fit Parameters:Export Tabulated Results", "Fluorescence Decay_Fit Parameters:MLE Baseline Offset Type", "Fluorescence Decay_Fit Parameters:MLE Baseline Offset", "Fluorescence Decay_Fit Parameters:Guess Parameter Names", "Fluorescence Decay_Fit Parameters:Guess Parameter Values", "Fluorescence Decay_Fit Parameters:Guess Parameters Options", "Fluorescence Decay_Fit Parameters:Optimal Offset Selection Criterion", "Fluorescence Decay_Styles:Show Last Decay Only", "Fluorescence Decay_Styles:Decay Graph Color Array", "Fluorescence Decay:Decay Graph Active", "Fluorescence Decay Statistics:Min Peak Value", "Fluorescence Decay Statistics:Reject Low Decay Peak Pixels", "Fluorescence Decay Statistics:Reject High Decay Peak Pixels", "Fluorescence Decay Statistics:Max Peak Value", "Time Traces:Use File Timestamp", "Time Traces:Time Step", "Time Traces:Use Intensity Correction File", "Time Traces:Intensity Correction File", "Phasor Plot:Phasor Plot Smoothing Options", "Phasor Plot:Phasor Plot Size", "Phasor Plot:Phasor Plot Graphics Options", "Phasor Plot:Cumulative Phasor Plot", "Phasor Plot:Use Phasor Brightness", "Phasor Plot:Blend Overlay with Phasor Background", "Phasor Plot:Save Phasor Plot", "Phasor Plot:Show References", "Phasor Plot:Phasor Ratio Decay Range", "Phasor Plot:Exponential Fading", "Phasor Plot:Phasor Ratio Reference Colors", "Phasor Plot:Reference Radius", "Phasor Plot:Show Color Map Vertices", "Phasor Plot:Phasor Plot Active", "Phasor Plot:Phasor Ratio Color Map Type", "Phasor Plot:Phasor Ratio Color Map", "Phasor Plot:Phasor Ratio Display Range", "Phasor Plot:Selected Image ROI(s)", "Phasor Plot:All Image ROIs", "Phasor Plot:Selected Phasor Plot ROI(s)", "Phasor Plot:All Phasor Plot ROIs", "Phasor Plot:Phasor Ratio Color-Coded Quantity", "Phasor Plot:Store Phasor Harmonics", "Phasor Plot:Draw Reference Segment", "Phasor Plot:User-Defined Quantity", "Phasor Plot:Color Scale High Color", "Phasor Plot:Color Scale Low Color", "Phasor Plot:Intensity-weighted Phasor Plot", "Phasor Graph:Phasor Frequency", "Phasor Graph:Phasor Ratio Type", "Phasor Graph:Pixel-level Phasor Computation", "Phasor Graph:Save Phasor Graph", "Phasor Graph:Phasor Graph Active", "Phasor Graph:Phasor SDV Options", "Phasor Graph:Intensity-weighted Phasor Graph", "Phasor Graph:Define Shortest Lifetime as", "Phasor Calibration:Use Backup Calibration if needed", "Phasor Calibration:Backup Calibration Type", "Phasor Calibration:Calibration Type", "Phasor Calibration:Calibration Lifetime", "Phasor Calibration:Calibration Map Algorithm", "Single-Exponential Phasor Locus (SEPL):Gate Parameters", "Single-Exponential Phasor Locus (SEPL):User-defined Gate", "Single-Exponential Phasor Locus (SEPL):User-defined IRF", "Single-Exponential Phasor Locus (SEPL):Phasor Parameters", "Single-Exponential Phasor Locus (SEPL):Decay & IRF Parameters", "Single-Exponential Phasor Locus (SEPL):Display Parameters", "Lifetime Analysis:Decay Analysis Parameters", "Lifetime Analysis:Lifetime Map Active", "Plugins:Python Settings", "Miscellaneous:Verbose Mode", "Miscellaneous:Beep after Script", "Miscellaneous:Saved Image File Format", "Miscellaneous:Exported Gate Image Settings", "Miscellaneous:Include Loading in Timing", "Miscellaneous:Verbose Settings Mode", "Miscellaneous:Histogram Options", "Miscellaneous:Beep on Error", "Miscellaneous:# Logical Processors Used", "Miscellaneous:ROI Description Max Characters", "Miscellaneous:Verbose Error Mode", "Miscellaneous:Transparent Mask Color"}
  T56 = typedef "AlliGator Action Engine.lvlib/Alligator Elements Order in Action Stack.ctl" = enum16{"Enqueue 2 AFTER 1", "Enqueue 2 BEFORE 1"}
  T57 = typedef "AlliGator Debug.lvlib/AlliGator Debug Action List.ctl" = enum16{"SS3 Gate Slip Correction", "Test Progress Bar", "Check Reference/IRF Definition", "Fit to Cubic Spline + Sine", "Check SS2 data scrambling", "Remove Image Outliers", "Test Python Plugin", "Edge ROI", "Change Frequency Programmatically", "Open Local Decay Graph Window", "Test Flatfield Correction", "Test Critical Bug", "Test Color Ramp Refnum"}
  T58 = typedef "AlliGator Action Engine.lvlib/AlliGator Q Element.ctl" = cluster{"AlliGator Q Event":T41, "Data":variant}
  T59 = typedef "AlliGator Action Engine.lvlib/AlliGator Event Category.ctl" = enum16{"GUI", "Files", "FLI Dataset", "FLI Dataset Series", "Image", "Decay", "Intensity Time Trace", "Phasor Plot", "Phasor Graph", "Phasor Ratio", "Lifetime", "Calibration", "Decay Fit Parameter Map", "Parameter Map", "Generic Graph", "DEBUG"}
  T60 = typedef "Notebook.lvlib/Notebook Message Object.ctl" = cluster{"Message":string, "Message Style":T61}
  T61 = typedef "Rich Text Box.lvlib/Text Formatting.ctl" = cluster{"Font":string, "Text Color":T62, "Background Color":T62, "Style":T63, "Font Size":dbl, "Alignment":T64}
  T62 = typedef "Rich Text Box.lvlib/Text Colors.ctl" = enum16{"Unchanged", "Black", "Blue", "Cyan", "Maroon", "Gray", "Violet", "Green", "Light Green", "Orange", "Yellow", "Magenta", "Red", "White"}
  T63 = typedef "Rich Text Box.lvlib/Text Style.ctl" = enum16{"Regular", "Bold", "Italic", "Underline", "Strikeout"}
  T64 = typedef "Rich Text Box.lvlib/Text Alignment.ctl" = enum16{"Left", "Right", "Center"}
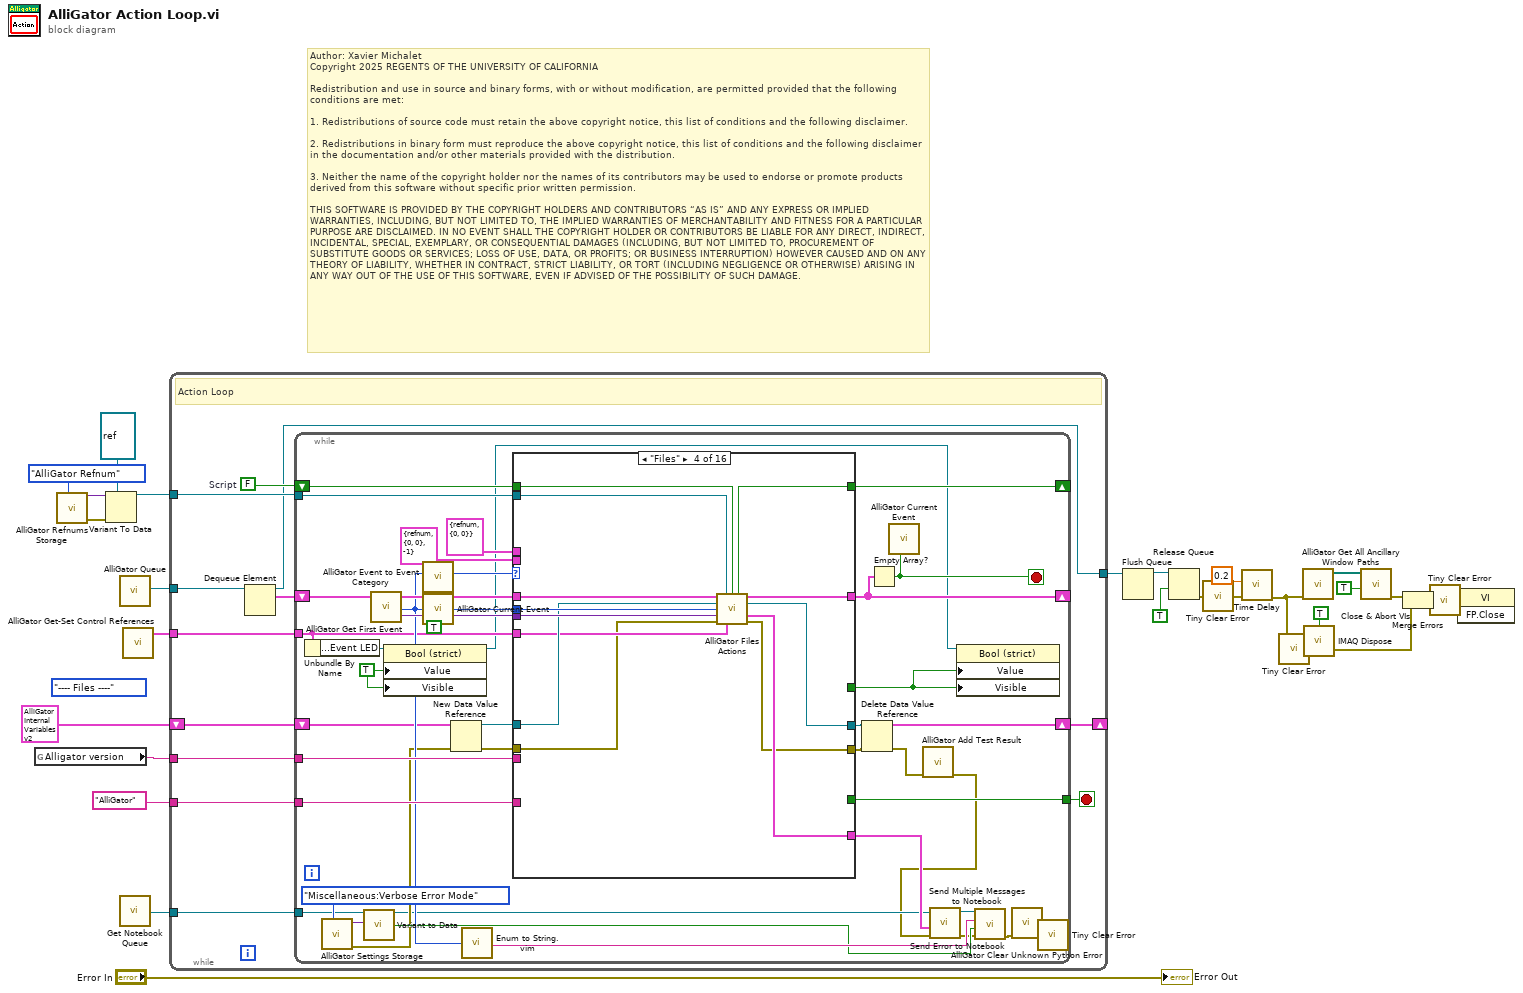
[diagram p0: block diagram]
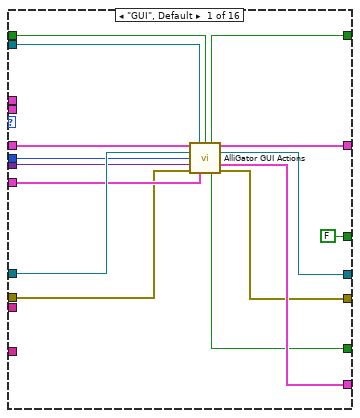
[diagram p2: hidden frame]
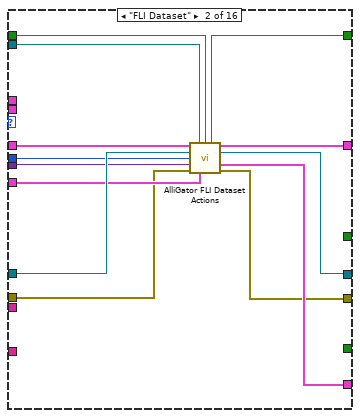
[diagram p3: hidden frame]
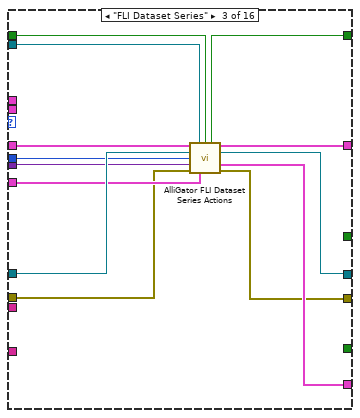
[diagram p4: hidden frame]
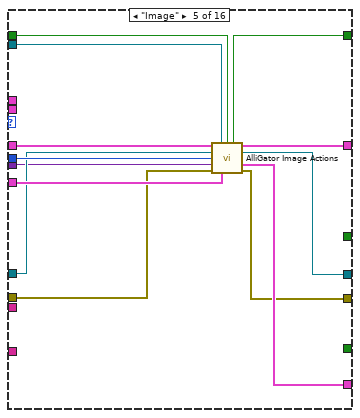
[diagram p5: hidden frame]
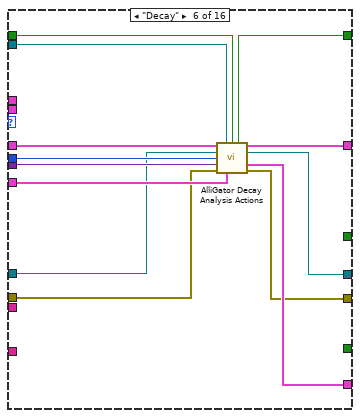
[diagram p6: hidden frame]
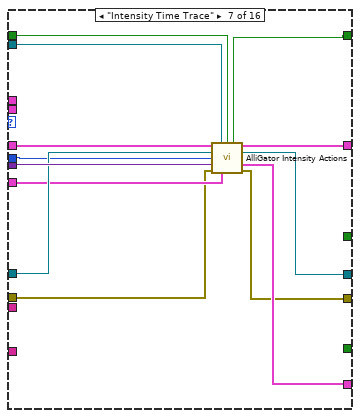
[diagram p7: hidden frame]
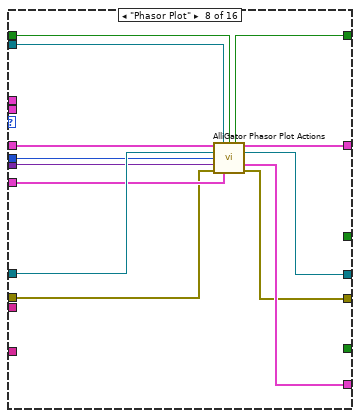
[diagram p8: hidden frame]
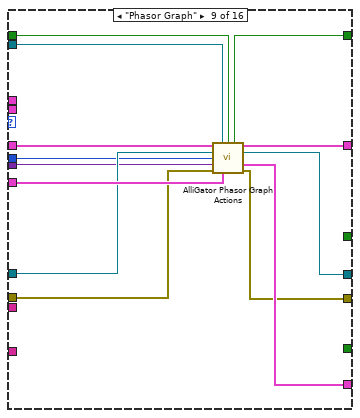
[diagram p9: hidden frame]
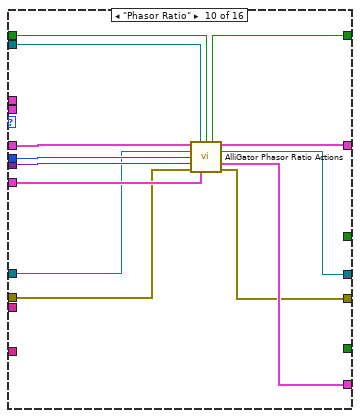
[diagram p10: hidden frame]
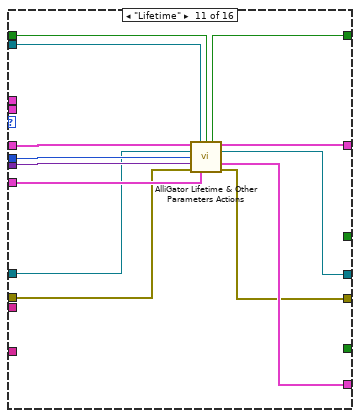
[diagram p11: hidden frame]
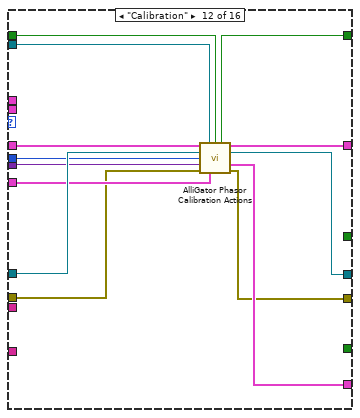
[diagram p12: hidden frame]
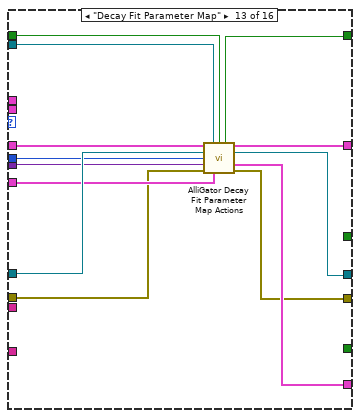
[diagram p13: hidden frame]
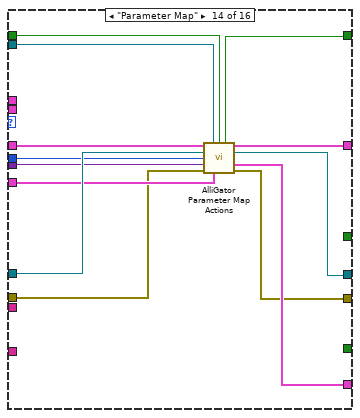
[diagram p14: hidden frame]
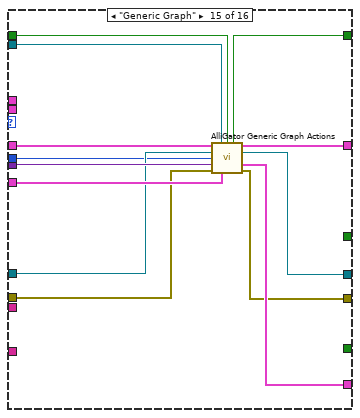
[diagram p15: hidden frame]
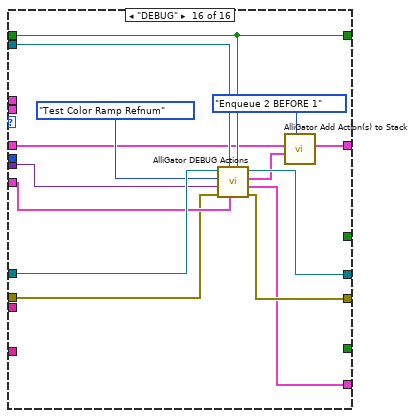
[diagram p16: hidden frame]
diagram:
  (unwired) AlliGator_Q_Event."---- Files ----" ("AlliGator Q Event out")
  # "Author: Xavier Michalet\nCopyright 2025 REGENTS OF THE UNIVERSITY OF CALIFORNIA\n\nRedistribution and use in source and binary forms, with or without modification, are permitted provided that the following conditions are met:\n\n1. Redistributions of source code must retain the above copyright notice, this list of conditions and the following disclaimer.\n\n2. Redistributions in binary form must reproduce the above copyright notice, this list of conditions and the following disclaimer in the documentation and/or other materials provided with the distribution.\n\n3. Neither the name of the copyright holder nor the names of its contributors may be used to endorse or promote products derived from this software without specific prior written permission.\n\nTHIS SOFTWARE IS PROVIDED BY THE COPYRIGHT HOLDERS AND CONTRIBUTORS “AS IS” AND ANY EXPRESS OR IMPLIED WARRANTIES, INCLUDING, BUT NOT LIMITED TO, THE IMPLIED WARRANTIES OF MERCHANTABILITY AND FITNESS FOR A PARTICULAR PURPOSE ARE DISCLAIMED. IN NO EVENT SHALL THE COPYRIGHT HOLDER OR CONTRIBUTORS BE LIABLE FOR ANY DIRECT, INDIRECT, INCIDENTAL, SPECIAL, EXEMPLARY, OR CONSEQUENTIAL DAMAGES (INCLUDING, BUT NOT LIMITED TO, PROCUREMENT OF SUBSTITUTE GOODS OR SERVICES; LOSS OF USE, DATA, OR PROFITS; OR BUSINESS INTERRUPTION) HOWEVER CAUSED AND ON ANY THEORY OF LIABILITY, WHETHER IN CONTRACT, STRICT LIABILITY, OR TORT (INCLUDING NEGLIGENCE OR OTHERWISE) ARISING IN ANY WAY OUT OF THE USE OF THIS SOFTWARE, EVEN IF ADVISED OF THE POSSIBILITY OF SUCH DAMAGE."
  n1 = global read "AlliGator Globals.vi" "Alligator version"() -> (w26:string)
  n2 = call "AlliGator Refnums Storage.vi"("AlliGator Refnum List"=AlliGator_Refnums_List."AlliGator Refnum") -> ("Error Out"=w4:errorcluster, "Data out"=w5:variant)  [unwired: 9 in]
  n3 = Variant To Data(error in=w4, type=refnum<vi> refnum ("AlliGator Refnum"), Variant=w5) -> (data=w2:refnum<vi>)  [unwired: 1 out]
  n4 = call "AlliGator Queue.vi"() -> ("AlliGator Q"=w10:refnum<queue>)  [unwired: 8 in, 1 out]
  n5 = call "Get Notebook Queue.vi"() -> ("Notebook Queue"=w25:refnum<queue>)  [unwired: 9 in]
  n6 = call "AlliGator Get-Set Control References.vi"() -> ("AlliGator Ctrl Refnums out"=w6:T42)  [unwired: 10 in, 1 out]
  n7 = while {
    tunnel: w2 -> [w38]
    tunnel: w25 -> [w37]
    shift-right: [w36] -> _
    shift-left: T2 {"----------------------------- Images -----------------------------"=0, "Displayed Image"=refnum, "White Light Image"=refnum, "Mask Image"=refnum, "ROI Mask Image"=refnum, "Current Dataset Images 1"={"SGL Gate Images"=[], "SGL Sum Image"=refnum, "SGL Max Image"=refnum, "SGL Min Image"=refnum}, "Background Dataset Images 1"={"SGL Gate Images"=[], "SGL Sum Image"=refnum, "SGL Max Image"=refnum, "SGL Min Image"=refnum}, "Current Dataset Images 2"={"SGL Gate Images"=[], "SGL Sum Image"=refnum, "SGL Max Image"=refnum, "SGL Min Image"=refnum}, "Background Dataset Images 2"={"SGL Gate Images"=[], "SGL Sum Image"=refnum, "SGL Max Image"=refnum, "SGL Min Image"=refnum}, "Current Dataset Arithmetic Images"={"SGL Gate Images"=[], "SGL Sum Image"=refnum, "SGL Max Image"=refnum, "SGL Min Image"=refnum}, "Accumulated Dataset Images 1"={"SGL Gate Images"=[], "SGL Sum Image"=refnum, "SGL Max Image"=refnum, "SGL Min Image"=refnum}, "Accumulated Dataset Images 2"={"SGL Gate Images"=[], "SGL Sum Image"=refnum, "SGL Max Image"=refnum, "SGL Min Image"=refnum}, "Accumulated Dataset Arithmetic Images"={"SGL Gate Images"=[], "SGL Sum Image"=refnum, "SGL Max Image"=refnum, "SGL Min Image"=refnum}, "----------------------------- File Paths -----------------------------"=0, "Phasor Plot Image"=refnum, "Decay Fit Parameter Map Image"=refnum, "Parameter Map Image"=refnum, "Single Data Point Path"=path "", "White Light Image Path"=path "", "Mask Image Path"=path "", "Time-Series Folder"=path "", "[Time-Series Paths]"=[], "----------------------------- FLI Dataset -----------------------------"=0, "Current Dataset"=0, "Single Dataset Type"=enum."HDF5 FLI Dataset", "Current Folder"="", "AlliGator Data Series Type"=enum."HDF5 FLI Dataset Series", "# Datasets"=0, "Dual-Channel Dataset"=FALSE, "Selected Channel Name"="", "Dataset Channel"=enum."G2", "Channel Arithmetic"=enum."None", "Dual-Channel Background Dataset"=FALSE, "Background Channel"=enum."G2", "Dual-Channel Accumulated Dataset"=FALSE, "Start Time"=0.0, "[Time-Series Timestamps]"=[], "[Intensity Corrections]"=[], "Time Series Script"=FALSE, "Type of Displayed Image"=enum."Sum of All Gates", "Gate Image Slide"=0, "# Gates"=0, "ROIs"=[], "----------------------------- Decays -----------------------------"=0, "ROI Decay"={"t Array"=[], "I Array"=[]}, "Valid Decay"=FALSE, "Decay  Metadata"={"ROI Descriptor"={"Global Rectangle"=[], "Contours"=[]}, "ROI Center"={"X"=0, "Y"=0}, "Decay Background Subtraction Info"={"Laser Period"=0.0, "Gate Duration"=0.0, "Baseline Subtraction Method"=enum."Mean", "Background Definition Range"={"Min Gate"=0.0, "Max Gate"=0.0}, "Total Intensity w/o Bkgd Subtraction"=0.0, "Bkgd-subtracted Intensity (exp)"=0.0, "# Data Points"=0, "Background/Gate"=0.0, "Fitted Lifetime"=0.0, "Bkgd-subtracted Intensity (theo)"=0.0}, "Decay Reverted"=FALSE, "Decay Smoothened"=FALSE, "Decay Straightened"=FALSE, "Fitted Tau (Decay Straightening)"=0.0, "Decay Shift Parameters"={"Type"=enum."Default", "Shift"=0.0, "Threshold"=0.0, "Rotate"=FALSE}, "Decay Shifted"=FALSE, "Decay Extrapolated"=FALSE, "Decay Extrapolation Parameters"={"Additional Points"=0, "Head Fraction"=0.0, "Fitted Tau"=0.0, "Use Periodicity"=FALSE, "Use Cursors"=FALSE, "Tail Fraction"=0.0}, "Decay Normalized"=FALSE, "Fold Decay"=FALSE, "# Folds"=1}, "Reference Decay Plot Name"="", "Reference Decay"={"t Array"=[], "I Array"=[]}, "Decay Shift Plot"={"Time Stamps"=[], "Decay Shifts"=[]}, "[Decays Max Values]"=[], "[Decays Min Values]"=[], "----------------------------- Calibration -----------------------------"=0, "Calibration Phasor"={"m"=0.0, "phi"=0.0, "Phasor Frequency"=0.0, "Reference Lifetime"=0.0}, "Calibration Phasor Series"={"m Array"=[], "phi Array"=[], "Phasor Frequency"=0.0, "Calibration Lifetime"=0.0}, "Phasor Calibration Map"={"Phasor Frequency"=80000000.0, "Calibration Lifetime"=1e-09, "ROI Centers"=[], "ROI Descriptors"=[], "Map Resolution X"=0, "Map Resolution Y"=0, "z Array"=[]}, "Calibration Map MD5 Digest"="", "----------------------------- Phasor Graph -----------------------------"=0, "Last Raw Phasor"={"g"=0.0, "s"=0.0}, "Last Calibrated Phasor"={"g"=0.0, "s"=0.0}, "Last Calibrated Phasor SDV"={"g"=0.0, "s"=0.0}, "Phasor Graph:Phasor Plot"={"g Array"=[], "s Array"=[]}, "Phasor Graph:Phasor SDV Plot"={"g Array"=[], "s Array"=[]}, "[Phasor Graph:Raw Phasor Plots]"=[], "Phasor Plot locked to Ref 1"=-1, "[Phasor Plot(s) locked to Ref 1]"=[], "[Phasor Plot(s) locked to Ref 2]"=[], "[Pixel Phasors]"=[], "----------------------------- Phasor Plot -----------------------------"=0, "[[Sum Image]]"=[], "[[CSG Phasors]]"=[], "[[Valid Pixel?]]"=[], "[[Phasor Ratios]]"=[], "[[Average Lifetimes]]"=[], "Amplitude Weighted Average Lifetime"=FALSE, "I/m/phi Dataset"={"I/m/phi Dataset?"=FALSE, "Base Frequency"=0.0, "Harmonic Orders"=[]}, "Multi Phasor Plot Data"={"Base Frequency"=0.0, "# Harmonics"=0, "Harmonic Orders"=[], "Phasor Plot Settings Checksum"=0, "Phasor Harmonic Data Array"=[]}, "----------------------------- Decay Fit Parameter Map -----------------------------"=0, "Decay Fit Options & Parameters"={"SYNC Period"=0.0, "Fit Options"={"Show Fit Residuals"=FALSE, "Fit Model"=enum."1-Exponential", "Residual Type"=enum."Standard", "Max Decay Percentile"=0.0, "Min Decay Percentile"=0.0, "Show Full Decay"=FALSE, "Weights"=enum."Unweighted", "Fitting Method"=enum."Least Square", "Compute Parameter Uncertainties"=FALSE, "Periodic Boundaries"=FALSE, "Model Calculation"=enum."Simulation", "Period"=0.0, "Termination Criteria"={"Max Iterations"=0, "Max Function Calls"=0, "Max Time"=0.0, "Function Tolerance"=0.0, "Parameter Tolerance"=0.0, "Gradient Tolerance"=0.0, "Min Lambda"=0.0, "Max Lambda"=0.0, "Initial Tick Count"=0}, "Offset Resolution"=0.0, "Use Local IRF"=FALSE, "Fitting Algorithm"=enum."Levenberg-Marquardt", "Show Confidence Interval "=TRUE, "Confidence Level"=95.0}, "Fit Parameter Constraints"=[], "MLE Baseline Offset"=0.0, "MLE Baseline Offset Type"=enum."Absolute"}, "Fit Options: Decay Preprocessing Parameters"={"Background Subtraction"=FALSE, "Straighten Decay"=FALSE, "Reverse Gates"=FALSE, "1-Normalized Decay"=FALSE, "Smoothen Decay"=FALSE, "Smoothing Parameter"=0.0, "Shift Decay"=FALSE, "Decay Shift Parameters"={"Type"=enum."Default", "Shift"=0.0, "Threshold"=0.0, "Rotate"=FALSE}, "Extrapolate Decay"=FALSE, "Additional Points"=0, "Head Fraction"=0.0, "Pixel-Normalize Decay"=FALSE, "Use Periodicity"=FALSE, "Use Cursors"=FALSE, "Tail Fraction"=0.0, "Use Decay Pre-Processing"=TRUE, "Fold Decay"=FALSE, "# Folds"=1, "[0-1]-Normalized Decay"=FALSE}, "Fit Options: Reference Decay"={"t Array"=[], "I Array"=[]}, "Is Full Image Parameters Map"=FALSE, "Is Single-Pixels Parameters Map"=FALSE, "NLSF Parameters Map X Resolution"=0, "NLSF Parameters Map Y Resolution"=0, "[Single Decay Fit Parameters]"=[], "Fit Model"=enum."1-Exponential", "[[Multiple Decays Fit Parameters]]"=[], "[[Multiple Decays Fit Parameter SDVs]]"=[], "[[IRFs]]"=[], "[ROI Descriptors]"=[], "IRF Array Time Axis"=[], "Decay Array Time Axis"=[], "[Decay Fit Parameter Names]"=[], "[Decay Sum]"=[], "Array of Decay Fit Result Constraints"=[], "Selected ROIs Array"=[], "----------------------------- Parameter Maps -----------------------------"=0, "[Map Set Names]"=[], "[Parameter Maps]"=[], "[[User-defined Quantities]]"=[], "User-defined Quantity"=""} ("AlliGator Internal Variables") -> [w30]
    tunnel: w26 -> [w35]
    tunnel: "AlliGator" ("Sender") -> [w33]
    tunnel: w6 -> [w32]
    tunnel: w10 -> [w28]
    tunnel: [w29] -> w14
    stop <- w31 stop-if-true
    w34 = FALSE  # Script
    # "Action Loop"
    n8 = Dequeue Element(queue=w28) -> (queue out=w29:refnum<queue>, element=w39:T58[])  [unwired: 2 in, 2 out]
    n9 = while {
      tunnel: [w44] -> w31
      shift-right: [w79] -> _
      shift-left: w39 -> [w74]
      tunnel: w38 -> [w76]
      tunnel: w37 -> [w41]
      shift-right: [w59] -> w36
      shift-left: w30 -> [w62]
      tunnel: w35 -> [w78]
      shift-right: [w58] -> _
      shift-left: w34 -> [w77]
      tunnel: w33 -> [w75]
      tunnel: w32 -> [w57]
      stop <- w66 stop-if-true
      w48 = TRUE ("Value")
      n10 = Unbundle By Name(w57) -> ("Other AlliGator Ctrl Refnums.Event LED"=w56:refnum<vi>)
      n11 = call "AlliGator Settings Storage.vi"("AlliGator Settings List"=AlliGator_Settings_List."Miscellaneous:Verbose Error Mode") -> ("Error Out"=w52:errorcluster, "Variant Data out"=w71:variant)  [unwired: 9 in]
      n12 = call-poly "Variant to Data.vi"("Variant"=w71) -> ("Value"=w54:bool)  [unwired: 8 in]
      n13 = call "AlliGator Get First Event.vi"("AlliGator Q Elements"=w74) -> ("Data"=w73:variant, "AlliGator Q Event"=w65:T41, "AlliGator Q Elements"=w80:T58[])  [unwired: 2 in]
      n14 = property class="Bool (strict)"(reference=w56, "Value"=w48, "Visible"=w48) -> (reference out=w45:refnum<vi>)  [unwired: 1 in, 1 out]
      n15 = call "AlliGator Event to Event Category.vi"("AlliGator Q Event"=w65) -> ("Event Category"=w68:T59)  [unwired: 8 in]
      n16 = call "AlliGator Current Event.vi"("AlliGator Q Event in"=w65, "Get(F)/Set"=TRUE) -> ("AlliGator Q Event out"=w63:T41)  [unwired: 7 in]
      n17 = New Data Value Reference(data value=w62, error in=w52) -> (data value reference=w61:refnum<data-value>, error out=w51:errorcluster)
      n18 = call "Enum to String.vim"("Enum"=w65) -> ("String"=w55:string)
      n19 = case shown="\"Files\"" w68 {
        tunnel: [FALSE ("Quit?") _ _ _ _ _ _ _ _ _ _ _ _ _ _ _] -> w49
        tunnel: w80 -> [w95 w108 w121 w134 w147 w154 w173 w184 w199 w206 w219 w235 w251 w264 w277 w282]
        tunnel: [w94 w107 w120 w133 w146 w153 w172 w183 w198 w204 w217 w238 w250 w263 w276 w280] -> w79
        tunnel: w78 -> [_ _ _ _ _ _ _ _ _ _ _ _ _ _ _ _]
        tunnel: w77 -> [w91 w104 w117 w127 w140 w160 w161 w178 w197 w212 w225 w230 w240 w253 w269 w285]
        tunnel: w76 -> [w89 w102 w115 w132 w145 w159 w171 w181 w191 w207 w220 w236 w247 w260 w275 w291]
        tunnel: w75 -> [_ _ _ _ _ _ _ _ _ _ _ _ _ _ _ _]
        tunnel: w73 -> [w87 w100 w113 w131 w139 w157 w170 w179 w193 w208 w221 w232 w245 w258 w274 w287]
        tunnel: T54 {"Multiplot XY Graph"=refnum, "Mouse Coordinates"={"Horizontal"=0, "Vertical"=0}, "Plot Index"=-1} ("Selected Plot Info") -> [_ _ _ _ _ _ _ _ _ _ _ _ _ _ _ _]
        tunnel: w57 -> [w86 w99 w112 w126 w144 w158 w167 w185 w196 w209 w222 w231 w244 w257 w273 w286]
        tunnel: T51 {"Multiplot XY Graph"=refnum, "Mouse Coordinates"={"Horizontal"=0, "Vertical"=0}} ("Mouse Click Event Data") -> [_ _ _ _ _ _ _ _ _ _ _ _ _ _ _ _]
        tunnel: w63 -> [w88 w101 w114 w130 w143 w156 w166 w180 w192 w210 w223 w233 w246 w259 w270 _]
        tunnel: w61 -> [w93 w106 w119 w129 w142 w151 w169 w186 w195 w205 w218 w237 w249 w262 w272 w290]
        tunnel: [w92 w105 w118 w128 w141 w152 w168 w182 w194 w203 w216 w234 w248 w261 w271 w289] -> w60
        tunnel: [w90 w103 w116 w125 w138 w155 w162 w174 w190 w211 w224 w226 w239 w252 w265 w285] -> w58
        tunnel: [w85 w98 w111 w124 w137 w150 w165 w177 w189 w202 w215 w229 w243 w256 w268 w278] -> w42
        tunnel: w51 -> [w84 w97 w110 w123 w136 w149 w164 w176 w188 w201 w214 w228 w242 w255 w267 w284]
        tunnel: [w83 w96 w109 w122 w135 w148 w163 w175 w187 w200 w213 w227 w241 w254 w266 w283] -> w50
        tunnel: [w82 _ _ _ _ _ _ _ _ _ _ _ _ _ _ _] -> w44
        frame "GUI", Default {
          n20 = call "AlliGator GUI Actions.vi"("AlliGator Q Elements in"=w95, "VI in"=w89, "Script"=w91, "AlliGator IV DVR"=w93, "AlliGator Q Event in"=w88, "Data"=w87, "error in (no error)"=w84, "AlliGator Ctrl Refnums"=w86) -> ("Script?"=w90:bool, "AlliGator Q Elements out"=w94:T58[], "AlliGator IV DVR"=w92:refnum<data-value>, "[Notebook Message]"=w85:T60[], "Quit?"=w82:bool, "error out"=w83:errorcluster)  [unwired: 2 in]
        }
        frame "FLI Dataset" {
          n21 = call "AlliGator FLI Dataset Actions.vi"("AlliGator Q Elements"=w108, "VI in"=w102, "Script in"=w104, "AlliGator IV DVR in"=w106, "AlliGator Q Event in"=w101, "Data"=w100, "error in (no error)"=w97, "AlliGator Ctrl Refnums"=w99) -> ("Script out"=w103:bool, "Alligator Queue Elements"=w107:T58[], "AlliGator IV DVR out"=w105:refnum<data-value>, "[Notebook Message]"=w98:T60[], "error out"=w96:errorcluster)  [unwired: 3 in]
        }
        frame "FLI Dataset Series" {
          n22 = call "AlliGator FLI Dataset Series Actions.vi"("AlliGator Q Elements"=w121, "VI in"=w115, "Script in"=w117, "AlliGator IV DVR in"=w119, "AlliGator Q Event in"=w114, "Data"=w113, "error in (no error)"=w110, "AlliGator Ctrl Refnums"=w112) -> ("Script out"=w116:bool, "Alligator Queue Elements"=w120:T58[], "AlliGator IV DVR out"=w118:refnum<data-value>, "[Notebook Message]"=w111:T60[], "error out"=w109:errorcluster)  [unwired: 3 in]
        }
        frame "Files" {
          n23 = call "AlliGator Files Actions.vi"("AlliGator Q Elements in"=w134, "VI in"=w132, "Script in"=w127, "AlliGator IV DVR"=w129, "AlliGator Q Event in"=w130, "Data"=w131, "error in (no error)"=w123, "AlliGator Ctrl Refnums"=w126) -> ("Script out"=w125:bool, "AlliGator Q Elements out"=w133:T58[], "AlliGator IV DVR"=w128:refnum<data-value>, "[Notebook Message]"=w124:T60[], "error out"=w122:errorcluster)  [unwired: 3 in]
        }
        frame "Image" {
          n24 = call "AlliGator Image Actions.vi"("AlliGator Q Elements"=w147, "VI in"=w145, "Script in"=w140, "AlliGator IV DVR in"=w142, "AlliGator Q Event in"=w143, "Data"=w139, "error in (no error)"=w136, "AlliGator Ctrl Refnums"=w144) -> ("Script out"=w138:bool, "Alligator Queue Elements"=w146:T58[], "AlliGator IV DVR out"=w141:refnum<data-value>, "[Notebook Message]"=w137:T60[], "error out"=w135:errorcluster)  [unwired: 3 in]
        }
        frame "Decay" {
          n25 = call "AlliGator Decay Analysis Actions.vi"("AlliGator Q Elements in"=w154, "VI in"=w159, "Script in"=w160, "AlliGator IV DVR in"=w151, "AlliGator Q Event in"=w156, "Data"=w157, "error in (no error)"=w149, "AlliGator Ctrl Refnums"=w158) -> ("Script off"=w155:bool, "AlliGator Q Elements out"=w153:T58[], "AlliGator IV DVR out"=w152:refnum<data-value>, "[Notebook Message]"=w150:T60[], "error out"=w148:errorcluster)  [unwired: 3 in]
        }
        frame "Intensity Time Trace" {
          n26 = call "AlliGator Intensity Actions.vi"("AlliGator Q Elements in"=w173, "VI in"=w171, "Script in"=w161, "AlliGator IV DVR in"=w169, "AlliGator Q Event in"=w166, "Data"=w170, "error in (no error)"=w164, "AlliGator Ctrl Refnums"=w167) -> ("Script out"=w162:bool, "AlliGator Q Elements out"=w172:T58[], "AlliGator IV DVR out"=w168:refnum<data-value>, "[Notebook Message]"=w165:T60[], "error out"=w163:errorcluster)  [unwired: 3 in]
        }
        frame "Phasor Plot" {
          n27 = call "AlliGator Phasor Plot Actions.vi"("AlliGator Q Elements in"=w184, "VI in"=w181, "Script in"=w178, "data value reference in"=w186, "AlliGator Q Event in"=w180, "Data"=w179, "error in (no error)"=w176, "AlliGator Ctrl Refnums"=w185) -> ("Script out"=w174:bool, "AlliGator Q Elements out"=w183:T58[], "Data Value Reference out"=w182:refnum<data-value>, "[Notebook Message]"=w177:T60[], "error out"=w175:errorcluster)  [unwired: 3 in]
        }
        frame "Phasor Graph" {
          n28 = call "AlliGator Phasor Graph Actions.vi"("AlliGator Q Elements in"=w199, "VI in"=w191, "Script in"=w197, "Data Value Reference in"=w195, "AlliGator Q Event in"=w192, "Data"=w193, "error in (no error)"=w188, "AlliGator Ctrl Refnums"=w196) -> ("Script out"=w190:bool, "AlliGator Q Elements out"=w198:T58[], "Data Value Reference out"=w194:refnum<data-value>, "[Notebook Message]"=w189:T60[], "error out"=w187:errorcluster)  [unwired: 3 in]
        }
        frame "Phasor Ratio" {
          n29 = call "AlliGator Phasor Ratio Actions.vi"("AlliGator Q Elements in"=w206, "VI in"=w207, "Script in"=w212, "data value reference in"=w205, "AlliGator Q Event in"=w210, "Data"=w208, "error in (no error)"=w201, "AlliGator Ctrl Refnums"=w209) -> ("Script out"=w211:bool, "AlliGator Q Elements out"=w204:T58[], "Data Value Reference out"=w203:refnum<data-value>, "[Notebook Message]"=w202:T60[], "error out"=w200:errorcluster)  [unwired: 3 in]
        }
        frame "Lifetime" {
          n30 = call "AlliGator Lifetime & Other Parameters Actions.vi"("AlliGator Q Elements in"=w219, "VI in"=w220, "Script in"=w225, "AlliGator IV DVR in"=w218, "AlliGator Q Event in"=w223, "Data"=w221, "error in (no error)"=w214, "AlliGator Ctrl Refnums"=w222) -> ("Script out"=w224:bool, "AlliGator Q Elements out"=w217:T58[], "AlliGator IV DVR out"=w216:refnum<data-value>, "[Notebook Message]"=w215:T60[], "error out"=w213:errorcluster)  [unwired: 3 in]
        }
        frame "Calibration" {
          n31 = call "AlliGator Phasor Calibration Actions.vi"("AlliGator Q Elements"=w235, "VI in"=w236, "Script in"=w230, "data value reference"=w237, "AlliGator Q Event in"=w233, "Data"=w232, "error in (no error)"=w228, "AlliGator Ctrl Refnums"=w231) -> ("Script out"=w226:bool, "Alligator Queue Element 1 (+ 2)"=w238:T58[], "AlliGator IV DVR"=w234:refnum<data-value>, "[Notebook Message]"=w229:T60[], "error out"=w227:errorcluster)  [unwired: 3 in]
        }
        frame "Decay Fit Parameter Map" {
          n32 = call "AlliGator Decay Fit Parameter Map Actions.vi"("AlliGator Q Elements in"=w251, "VI in"=w247, "Script in"=w240, "data value reference"=w249, "AlliGator Q Event in"=w246, "Data"=w245, "error in (no error)"=w242, "AlliGator Ctrl Refnums"=w244) -> ("Script out"=w239:bool, "AlliGator Q Elements out"=w250:T58[], "Data Value Reference out"=w248:refnum<data-value>, "[Notebook Message]"=w243:T60[], "error out"=w241:errorcluster)  [unwired: 3 in]
        }
        frame "Parameter Map" {
          n33 = call "AlliGator Parameter Map Actions.vi"("AlliGator Q Elements in"=w264, "VI in"=w260, "Script in"=w253, "data value reference"=w262, "AlliGator Q Event in"=w259, "Data"=w258, "error in (no error)"=w255, "AlliGator Ctrl Refnums"=w257) -> ("Script out"=w252:bool, "AlliGator Q Elements out"=w263:T58[], "Data Value Reference out"=w261:refnum<data-value>, "[Notebook Message]"=w256:T60[], "error out"=w254:errorcluster)  [unwired: 3 in]
        }
        frame "Generic Graph" {
          n34 = call "AlliGator Generic Graph Actions.vi"("AlliGator Q Elements in"=w277, "VI in"=w275, "Script"=w269, "data value reference in"=w272, "AlliGator Q Event in"=w270, "Data"=w274, "error in (no error)"=w267, "AlliGator Ctrl Refnums"=w273) -> ("Script out"=w265:bool, "AlliGator Q Elements out"=w276:T58[], "Data Value Reference out"=w271:refnum<data-value>, "[Notebook Message]"=w268:T60[], "error out"=w266:errorcluster)  [unwired: 3 in]
        }
        frame "DEBUG" {
          n35 = call "AlliGator DEBUG Actions.vi"("Script"=w285, "AlliGator Ctrl Refnums"=w286, "VI in"=w291, "Error In"=w284, "Data"=w287, "Debug Action List"=AlliGator_Debug_Action_List."Test Color Ramp Refnum", "data value reference"=w290) -> ("Error Out"=w283:errorcluster, "[Notebook Message]"=w278:T60[], "AlliGator Action"=w281:T58[], "Data Value Reference out"=w289:refnum<data-value>)  [unwired: 1 in]
          n36 = call-poly "AlliGator Add Action(s) to Stack.vi"("Elements Order in Action Stack (Default: 2 BEFORE 1)"=Alligator_Elements_Order_in_Action_Stack."Enqueue 2 BEFORE 1", "Alligator Queue Element 2"=w281, "Alligator Queue Element 1"=w282) -> ("Alligator Queue Element 1 (+ 2)"=w280:T58[])  [unwired: 7 in, 1 out]
        }
      }
      n37 = Delete Data Value Reference(data value reference=w60, error in=w50) -> (data value=w59:T2, error out=w43:errorcluster)
      n38 = Empty Array?(array=w79) -> (empty?=w66:bool)
      n39 = call "AlliGator Current Event.vi"("Get(F)/Set"=w66) -> ()  [unwired: 8 in, 1 out]
      n40 = call "AlliGator Add Test Result.vi"("error in (no error)"=w43) -> ("error out"=w40:errorcluster)  [unwired: 10 in]
      n41 = call "Send Multiple Messages to Notebook.vi"("Error In"=w40, "[Notebook Message]"=w42, "Notebook Queue"=w41) -> ("Error Out"=w46:errorcluster, "Notebook Queue"=w47:refnum<queue>)  [unwired: 5 in]
      n42 = property class="Bool (strict)"(reference=w45, "Value"=w49, "Visible"=w49) -> ()  [unwired: 1 in, 2 out]
      n43 = call "Send Error to Notebook.vi"("error in (no error)"=w46, "Verbose Error Messages (T)"=w54, "State Machine Case Error Source"=w55, "Notebook Q"=w47) -> ("Error Out"=w69:errorcluster)  [unwired: 7 in]
      n44 = call "AlliGator Clear Unknown Python Error.vi"("error in (no error)"=w69) -> ("error out"=w53:errorcluster)  [unwired: 10 in]
      n45 = call "Tiny Clear Error.vi"("Error In"=w53) -> ()  [unwired: 8 in, 1 out]
    }
  }
  n46 = Flush Queue(queue=w14) -> (queue out=w13:refnum<queue>)  [unwired: 1 in, 2 out]
  n47 = Release Queue(queue=w13, force destroy? (F)=TRUE) -> (error out=w11:errorcluster)  [unwired: 1 in, 2 out]
  n48 = call "Tiny Clear Error.vi"("Error In"=w11) -> ("no Error Out"=w9:errorcluster)  [unwired: 8 in]
  n49 = call "Time Delay"("error in (no error)"=w9, "Delay Time (s)"=0.2 ("milliseconds to wait")) -> ("error out"=w8:errorcluster)  [unwired: 9 in]
  n50 = call "Tiny Clear Error.vi"("Error In"=w8) -> ("no Error Out"=w15:errorcluster)  [unwired: 8 in]
  n51 = call "AlliGator Get All Ancillary Window Paths.vi"("Error In"=w8) -> ("AlliGator Window Paths"=w23:path[])  [unwired: 9 in, 1 out]
  n52 = call "IMAQ Dispose"("All Images? (No)"=TRUE, "error in (no error)"=w15) -> ("error out"=w19:errorcluster)  [unwired: 4 in]
  n53 = call "Close & Abort VIs.vi"("Abort (T)"=TRUE, "VI Paths"=w23) -> ("Error Out"=w22:errorcluster)  [unwired: 9 in]
  n54 = Merge Errors(w22, w19) -> (w20:errorcluster)
  n55 = call "Tiny Clear Error.vi"("Error In"=w20) -> ("no Error Out"=w18:errorcluster)  [unwired: 8 in]
  n56 = invoke class="VI" method="FP.Close"(error in=w18) -> ()  [unwired: 2 in, 3 out]
  "Error Out" <- "Error In"
